vi "Open_Create File.vi"(8 "error in (no error)":errorcluster, 11 "TXT in":refnum<class "TXT.lvclass">) -> (0 "error out":errorcluster, 1 "Operation":T1, 2 "Path":path, 3 "TXT out":refnum<class "TXT.lvclass">)   [LabVIEW 2020, in "TXT.lvlib" / "TXT.lvclass"]
uses:
  TXT.lvclass
  built/windows/ImportExport.lvlibp/Operation.ctl
  TXT.lvclass/TXT.ctl
  built/windows/ImportExport.lvlibp/ConfigFile/ConfigFile.lvclass
  built/windows/ImportExport.lvlibp
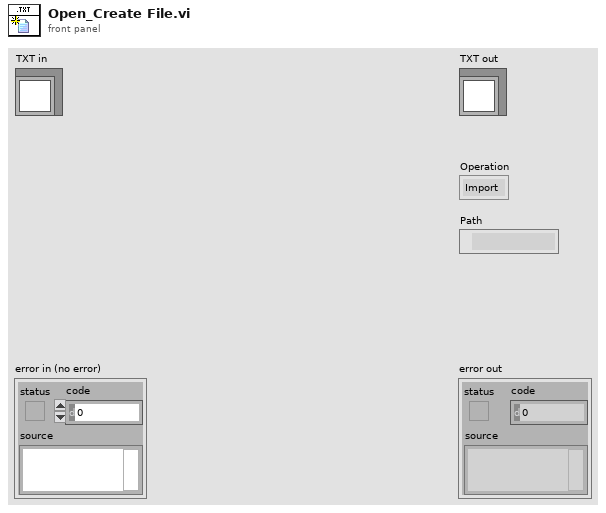
[diagram p1: front panel]
types:
  T1 = typedef "ImportExport.lvlibp/Operation.ctl" = enum16{"Import", "Export"}
  T2 = enum16{"open", "replace", "create", "open or create", "replace or create", "replace or create with confirmation"}
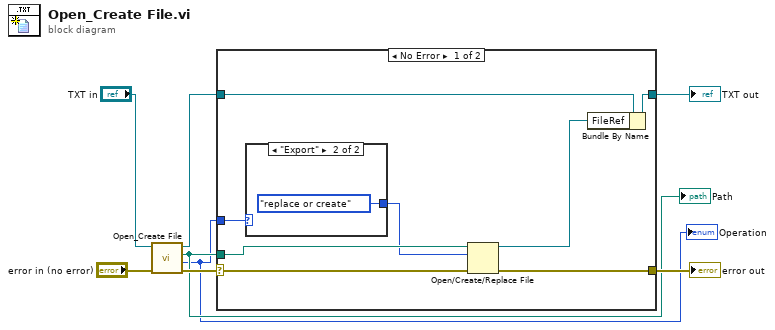
[diagram p0: block diagram]
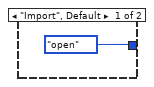
[diagram p2: hidden frame]
diagram:
  n1 = call-parent "Open_Create File.vi"("error in (no error)"="error in (no error)", "ConfigFile in"="TXT in") -> ("error out"=w5:errorcluster, "Operation"=w1:T1, "Path"=w2:path, "ConfigFile out"=w6:refnum<class "TXT.lvclass">)  [unwired: 6 in]
  "Path" <- w2
  "Operation" <- w1
  n2 = case shown="No Error" w5 {
    selector: w5 -> [w15 w20]
    tunnel: w6 -> [w12 w19]
    tunnel: [w14 w20] -> w4
    tunnel: [w16 w19] -> w3
    tunnel: w2 -> [w11 _]
    tunnel: w1 -> [w10 _]
    frame No Error {
      n3 = case shown="\"Export\"" w10 {
        tunnel: [T2."open" ("operation (0:open)") T2."replace or create" ("operation (0:open)")] -> w9
        frame "Import", Default {
        }
        frame "Export" {
        }
      }
      n4 = Open/Create/Replace File(file path (use dialog)=w11, error in=w15, operation (0:open)=w9) -> (refnum out=w13:refnum<file>, error out=w14:errorcluster)  [unwired: 3 in, 1 out]
      n5 = Bundle By Name(cluster=w12, "FileRef"=w13) -> (w16:refnum<class "TXT.lvclass">)
    }
    frame Error {
    }
  }
  "error out" <- w4
  "TXT out" <- w3
